vi "Sorting by.vi"(1 "Queue":T1(array[cluster])=[{"Measure?"=TRUE, "Area (cm^2)"=0.0, "Cell Label"="", "Cell Description"="", "Cell Position"=0, "Time in rig (h)"=0.0, "Time to next scan (min)"=0.0, "Scan number"=0.0, "When did you stick it in?"=0.0, "Time between scans (min)"=0.0, "Time of the last scan(min)"=0.0, "Scan settings in queue"=0}, {"Measure?"=TRUE, "Area (cm^2)"=0.0, "Cell Label"="", "Cell Description"="", "Cell Position"=0, "Time in rig (h)"=0.0, "Time to next scan (min)"=0.0, "Scan number"=0.0, "When did you stick it in?"=0.0, "Time between scans (min)"=0.0, "Time of the last scan(min)"=0.0, "Scan settings in queue"=0}, {"Measure?"=TRUE, "Area (cm^2)"=0.0, "Cell Label"="", "Cell Description"="", "Cell Position"=0, "Time in rig (h)"=0.0, "Time to next scan (min)"=0.0, "Scan number"=0.0, "When did you stick it in?"=0.0, "Time between scans (min)"=0.0, "Time of the last scan(min)"=0.0, "Scan settings in queue"=0}, {"Measure?"=TRUE, "Area (cm^2)"=0.0, "Cell Label"="", "Cell Description"="", "Cell Position"=0, "Time in rig (h)"=0.0, "Time to next scan (min)"=0.0, "Scan number"=0.0, "When did you stick it in?"=0.0, "Time between scans (min)"=0.0, "Time of the last scan(min)"=0.0, "Scan settings in queue"=0}, {"Measure?"=TRUE, "Area (cm^2)"=0.0, "Cell Label"="", "Cell Description"="", "Cell Position"=0, "Time in rig (h)"=0.0, "Time to next scan (min)"=0.0, "Scan number"=0.0, "When did you stick it in?"=0.0, "Time between scans (min)"=0.0, "Time of the last scan(min)"=0.0, "Scan settings in queue"=0}, {"Measure?"=TRUE, "Area (cm^2)"=0.0, "Cell Label"="", "Cell Description"="", "Cell Position"=0, "Time in rig (h)"=0.0, "Time to next scan (min)"=0.0, "Scan number"=0.0, "When did you stick it in?"=0.0, "Time between scans (min)"=0.0, "Time of the last scan(min)"=0.0, "Scan settings in queue"=0}, {"Measure?"=TRUE, "Area (cm^2)"=0.0, "Cell Label"="", "Cell Description"="", "Cell Position"=0, "Time in rig (h)"=0.0, "Time to next scan (min)"=0.0, "Scan number"=0.0, "When did you stick it in?"=0.0, "Time between scans (min)"=0.0, "Time of the last scan(min)"=0.0, "Scan settings in queue"=0}, {"Measure?"=TRUE, "Area (cm^2)"=0.0, "Cell Label"="", "Cell Description"="", "Cell Position"=0, "Time in rig (h)"=0.0, "Time to next scan (min)"=0.0, "Scan number"=0.0, "When did you stick it in?"=0.0, "Time between scans (min)"=0.0, "Time of the last scan(min)"=0.0, "Scan settings in queue"=0}, {"Measure?"=TRUE, "Area (cm^2)"=0.0, "Cell Label"="", "Cell Description"="", "Cell Position"=0, "Time in rig (h)"=0.0, "Time to next scan (min)"=0.0, "Scan number"=0.0, "When did you stick it in?"=0.0, "Time between scans (min)"=0.0, "Time of the last scan(min)"=0.0, "Scan settings in queue"=0}, {"Measure?"=TRUE, "Area (cm^2)"=0.0, "Cell Label"="", "Cell Description"="", "Cell Position"=0, "Time in rig (h)"=0.0, "Time to next scan (min)"=0.0, "Scan number"=0.0, "When did you stick it in?"=0.0, "Time between scans (min)"=0.0, "Time of the last scan(min)"=0.0, "Scan settings in queue"=0}, {"Measure?"=TRUE, "Area (cm^2)"=0.0, "Cell Label"="", "Cell Description"="", "Cell Position"=0, "Time in rig (h)"=0.0, "Time to next scan (min)"=0.0, "Scan number"=0.0, "When did you stick it in?"=0.0, "Time between scans (min)"=0.0, "Time of the last scan(min)"=0.0, "Scan settings in queue"=0}, {"Measure?"=TRUE, "Area (cm^2)"=0.0, "Cell Label"="", "Cell Description"="", "Cell Position"=0, "Time in rig (h)"=0.0, "Time to next scan (min)"=0.0, "Scan number"=0.0, "When did you stick it in?"=0.0, "Time between scans (min)"=0.0, "Time of the last scan(min)"=0.0, "Scan settings in queue"=0}, {"Measure?"=TRUE, "Area (cm^2)"=0.0, "Cell Label"="", "Cell Description"="", "Cell Position"=0, "Time in rig (h)"=0.0, "Time to next scan (min)"=0.0, "Scan number"=0.0, "When did you stick it in?"=0.0, "Time between scans (min)"=0.0, "Time of the last scan(min)"=0.0, "Scan settings in queue"=0}, {"Measure?"=TRUE, "Area (cm^2)"=0.0, "Cell Label"="", "Cell Description"="", "Cell Position"=0, "Time in rig (h)"=0.0, "Time to next scan (min)"=0.0, "Scan number"=0.0, "When did you stick it in?"=0.0, "Time between scans (min)"=0.0, "Time of the last scan(min)"=0.0, "Scan settings in queue"=0}, {"Measure?"=TRUE, "Area (cm^2)"=0.0, "Cell Label"="", "Cell Description"="", "Cell Position"=0, "Time in rig (h)"=0.0, "Time to next scan (min)"=0.0, "Scan number"=0.0, "When did you stick it in?"=0.0, "Time between scans (min)"=0.0, "Time of the last scan(min)"=0.0, "Scan settings in queue"=0}, {"Measure?"=TRUE, "Area (cm^2)"=0.0, "Cell Label"="", "Cell Description"="", "Cell Position"=0, "Time in rig (h)"=0.0, "Time to next scan (min)"=0.0, "Scan number"=0.0, "When did you stick it in?"=0.0, "Time between scans (min)"=0.0, "Time of the last scan(min)"=0.0, "Scan settings in queue"=0}] {"Scan settings in queue" items=["Regular", "Inverted"]; "Time of the last scan(min)" format="%<%H:%M:%S>t"; "When did you stick it in?" format="%<%H:%M:%S>t"; "Time to next scan (min)" format="%<%H:%M:%S>t"; "Time in rig (h)" format="%<%H:%M:%S>t"}, 2 "Sort by":u16(ring) items=["Cell position", "Cell label", "Time in rig"]) -> (0 "Queue 2":T1(array[cluster])=[{"Measure?"=TRUE, "Area (cm^2)"=0.0, "Cell Label"="", "Cell Description"="", "Cell Position"=0, "Time in rig (h)"=0.0, "Time to next scan (min)"=0.0, "Scan number"=0.0, "When did you stick it in?"=0.0, "Time between scans (min)"=0.0, "Time of the last scan(min)"=0.0, "Scan settings in queue"=0}, {"Measure?"=TRUE, "Area (cm^2)"=0.0, "Cell Label"="", "Cell Description"="", "Cell Position"=0, "Time in rig (h)"=0.0, "Time to next scan (min)"=0.0, "Scan number"=0.0, "When did you stick it in?"=0.0, "Time between scans (min)"=0.0, "Time of the last scan(min)"=0.0, "Scan settings in queue"=0}, {"Measure?"=TRUE, "Area (cm^2)"=0.0, "Cell Label"="", "Cell Description"="", "Cell Position"=0, "Time in rig (h)"=0.0, "Time to next scan (min)"=0.0, "Scan number"=0.0, "When did you stick it in?"=0.0, "Time between scans (min)"=0.0, "Time of the last scan(min)"=0.0, "Scan settings in queue"=0}, {"Measure?"=TRUE, "Area (cm^2)"=0.0, "Cell Label"="", "Cell Description"="", "Cell Position"=0, "Time in rig (h)"=0.0, "Time to next scan (min)"=0.0, "Scan number"=0.0, "When did you stick it in?"=0.0, "Time between scans (min)"=0.0, "Time of the last scan(min)"=0.0, "Scan settings in queue"=0}, {"Measure?"=TRUE, "Area (cm^2)"=0.0, "Cell Label"="", "Cell Description"="", "Cell Position"=0, "Time in rig (h)"=0.0, "Time to next scan (min)"=0.0, "Scan number"=0.0, "When did you stick it in?"=0.0, "Time between scans (min)"=0.0, "Time of the last scan(min)"=0.0, "Scan settings in queue"=0}, {"Measure?"=TRUE, "Area (cm^2)"=0.0, "Cell Label"="", "Cell Description"="", "Cell Position"=0, "Time in rig (h)"=0.0, "Time to next scan (min)"=0.0, "Scan number"=0.0, "When did you stick it in?"=0.0, "Time between scans (min)"=0.0, "Time of the last scan(min)"=0.0, "Scan settings in queue"=0}, {"Measure?"=TRUE, "Area (cm^2)"=0.0, "Cell Label"="", "Cell Description"="", "Cell Position"=0, "Time in rig (h)"=0.0, "Time to next scan (min)"=0.0, "Scan number"=0.0, "When did you stick it in?"=0.0, "Time between scans (min)"=0.0, "Time of the last scan(min)"=0.0, "Scan settings in queue"=0}, {"Measure?"=TRUE, "Area (cm^2)"=0.0, "Cell Label"="", "Cell Description"="", "Cell Position"=0, "Time in rig (h)"=0.0, "Time to next scan (min)"=0.0, "Scan number"=0.0, "When did you stick it in?"=0.0, "Time between scans (min)"=0.0, "Time of the last scan(min)"=0.0, "Scan settings in queue"=0}, {"Measure?"=TRUE, "Area (cm^2)"=0.0, "Cell Label"="", "Cell Description"="", "Cell Position"=0, "Time in rig (h)"=0.0, "Time to next scan (min)"=0.0, "Scan number"=0.0, "When did you stick it in?"=0.0, "Time between scans (min)"=0.0, "Time of the last scan(min)"=0.0, "Scan settings in queue"=0}, {"Measure?"=TRUE, "Area (cm^2)"=0.0, "Cell Label"="", "Cell Description"="", "Cell Position"=0, "Time in rig (h)"=0.0, "Time to next scan (min)"=0.0, "Scan number"=0.0, "When did you stick it in?"=0.0, "Time between scans (min)"=0.0, "Time of the last scan(min)"=0.0, "Scan settings in queue"=0}, {"Measure?"=TRUE, "Area (cm^2)"=0.0, "Cell Label"="", "Cell Description"="", "Cell Position"=0, "Time in rig (h)"=0.0, "Time to next scan (min)"=0.0, "Scan number"=0.0, "When did you stick it in?"=0.0, "Time between scans (min)"=0.0, "Time of the last scan(min)"=0.0, "Scan settings in queue"=0}, {"Measure?"=TRUE, "Area (cm^2)"=0.0, "Cell Label"="", "Cell Description"="", "Cell Position"=0, "Time in rig (h)"=0.0, "Time to next scan (min)"=0.0, "Scan number"=0.0, "When did you stick it in?"=0.0, "Time between scans (min)"=0.0, "Time of the last scan(min)"=0.0, "Scan settings in queue"=0}, {"Measure?"=TRUE, "Area (cm^2)"=0.0, "Cell Label"="", "Cell Description"="", "Cell Position"=0, "Time in rig (h)"=0.0, "Time to next scan (min)"=0.0, "Scan number"=0.0, "When did you stick it in?"=0.0, "Time between scans (min)"=0.0, "Time of the last scan(min)"=0.0, "Scan settings in queue"=0}, {"Measure?"=TRUE, "Area (cm^2)"=0.0, "Cell Label"="", "Cell Description"="", "Cell Position"=0, "Time in rig (h)"=0.0, "Time to next scan (min)"=0.0, "Scan number"=0.0, "When did you stick it in?"=0.0, "Time between scans (min)"=0.0, "Time of the last scan(min)"=0.0, "Scan settings in queue"=0}, {"Measure?"=TRUE, "Area (cm^2)"=0.0, "Cell Label"="", "Cell Description"="", "Cell Position"=0, "Time in rig (h)"=0.0, "Time to next scan (min)"=0.0, "Scan number"=0.0, "When did you stick it in?"=0.0, "Time between scans (min)"=0.0, "Time of the last scan(min)"=0.0, "Scan settings in queue"=0}, {"Measure?"=TRUE, "Area (cm^2)"=0.0, "Cell Label"="", "Cell Description"="", "Cell Position"=0, "Time in rig (h)"=0.0, "Time to next scan (min)"=0.0, "Scan number"=0.0, "When did you stick it in?"=0.0, "Time between scans (min)"=0.0, "Time of the last scan(min)"=0.0, "Scan settings in queue"=0}] {"Scan settings in queue" items=["Regular", "Inverted"]; "Time of the last scan(min)" format="%<%H:%M:%S>t"; "When did you stick it in?" format="%<%H:%M:%S>t"; "Time to next scan (min)" format="%<%H:%M:%S>t"; "Time in rig (h)" format="%<%H:%M:%S>t"})   [LabVIEW 2011]
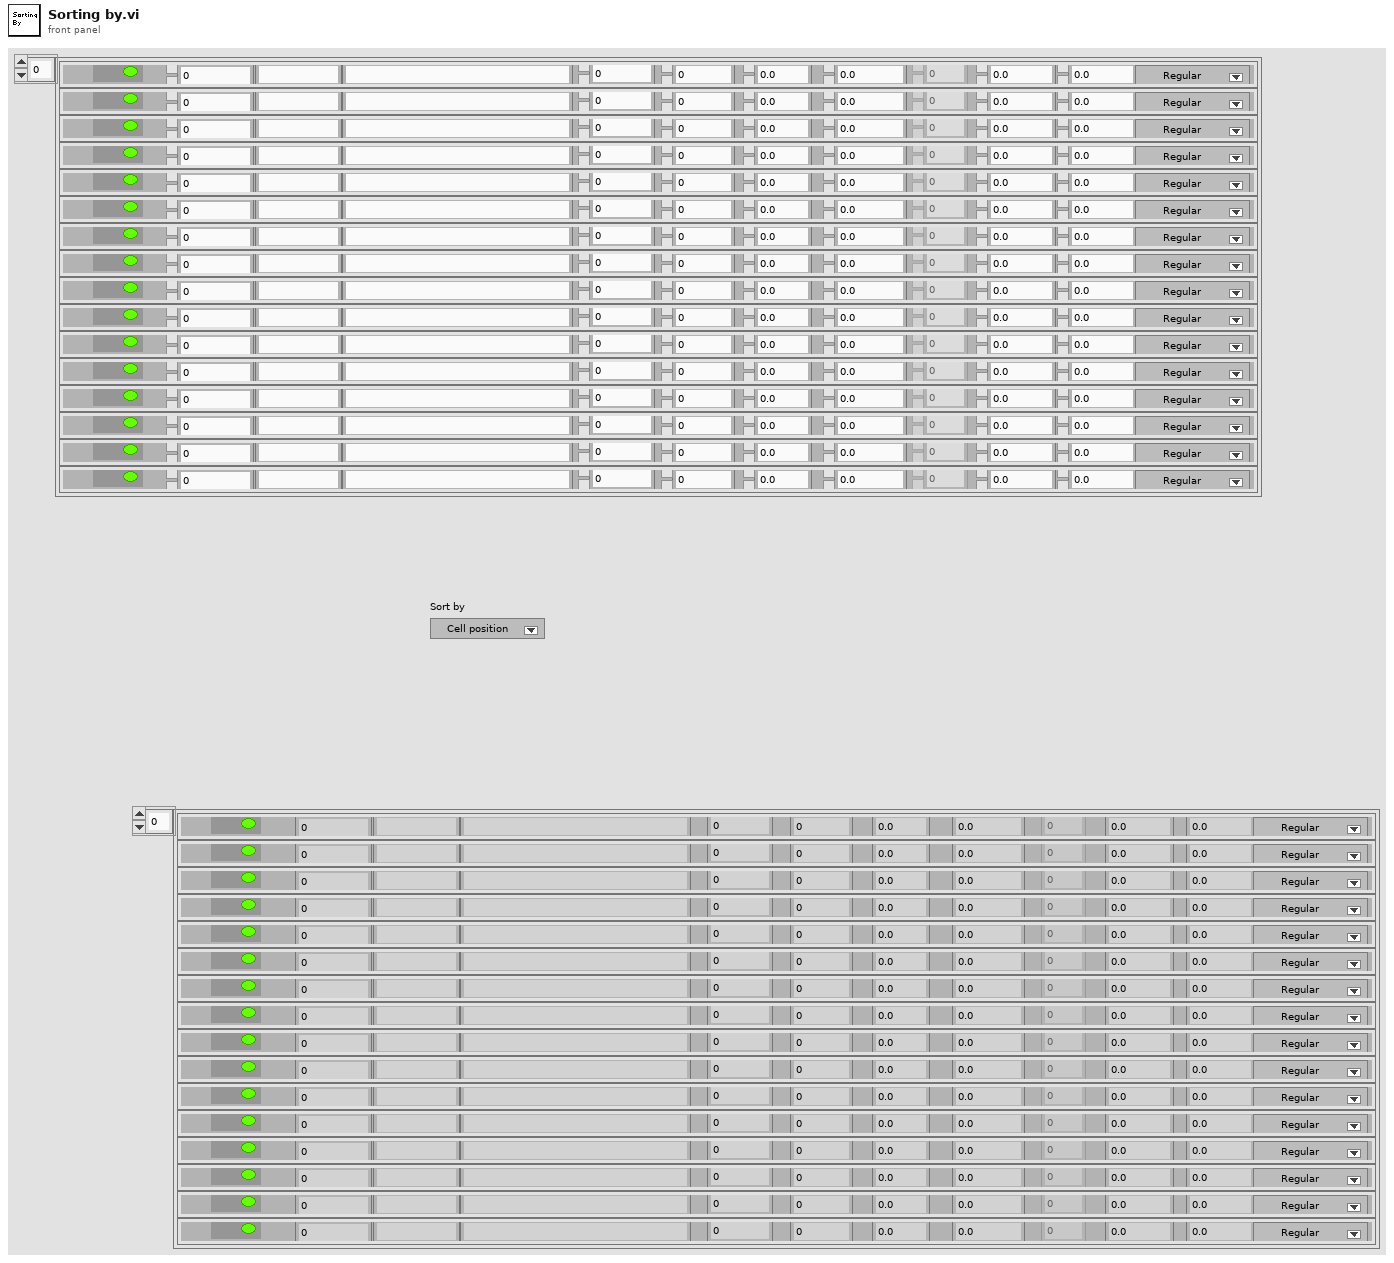
[diagram p1: front panel]
types:
  T1 = cluster{"Measure?":bool, "Area (cm^2)":dbl, "Cell Label":string, "Cell Description":string, "Cell Position":i32, "Time in rig (h)":dbl, "Time to next scan (min)":dbl, "Scan number":dbl, "When did you stick it in?":dbl, "Time between scans (min)":dbl, "Time of the last scan(min)":dbl, "Scan settings in queue":u16}[]
  T2 = cluster{"Measure?":bool, "Area (cm^2)":dbl, "Cell Label":string, "Cell Description":string, "Cell Position":i32, "Time in rig (h)":dbl, "Time to next scan (min)":dbl, "Scan number":dbl, "When did you stick it in?":dbl, "Time between scans (min)":dbl, "Time of the last scan(min)":dbl, "Scan settings in queue":u16}
  T3 = cluster{"cell label":string, "cell position":dbl}
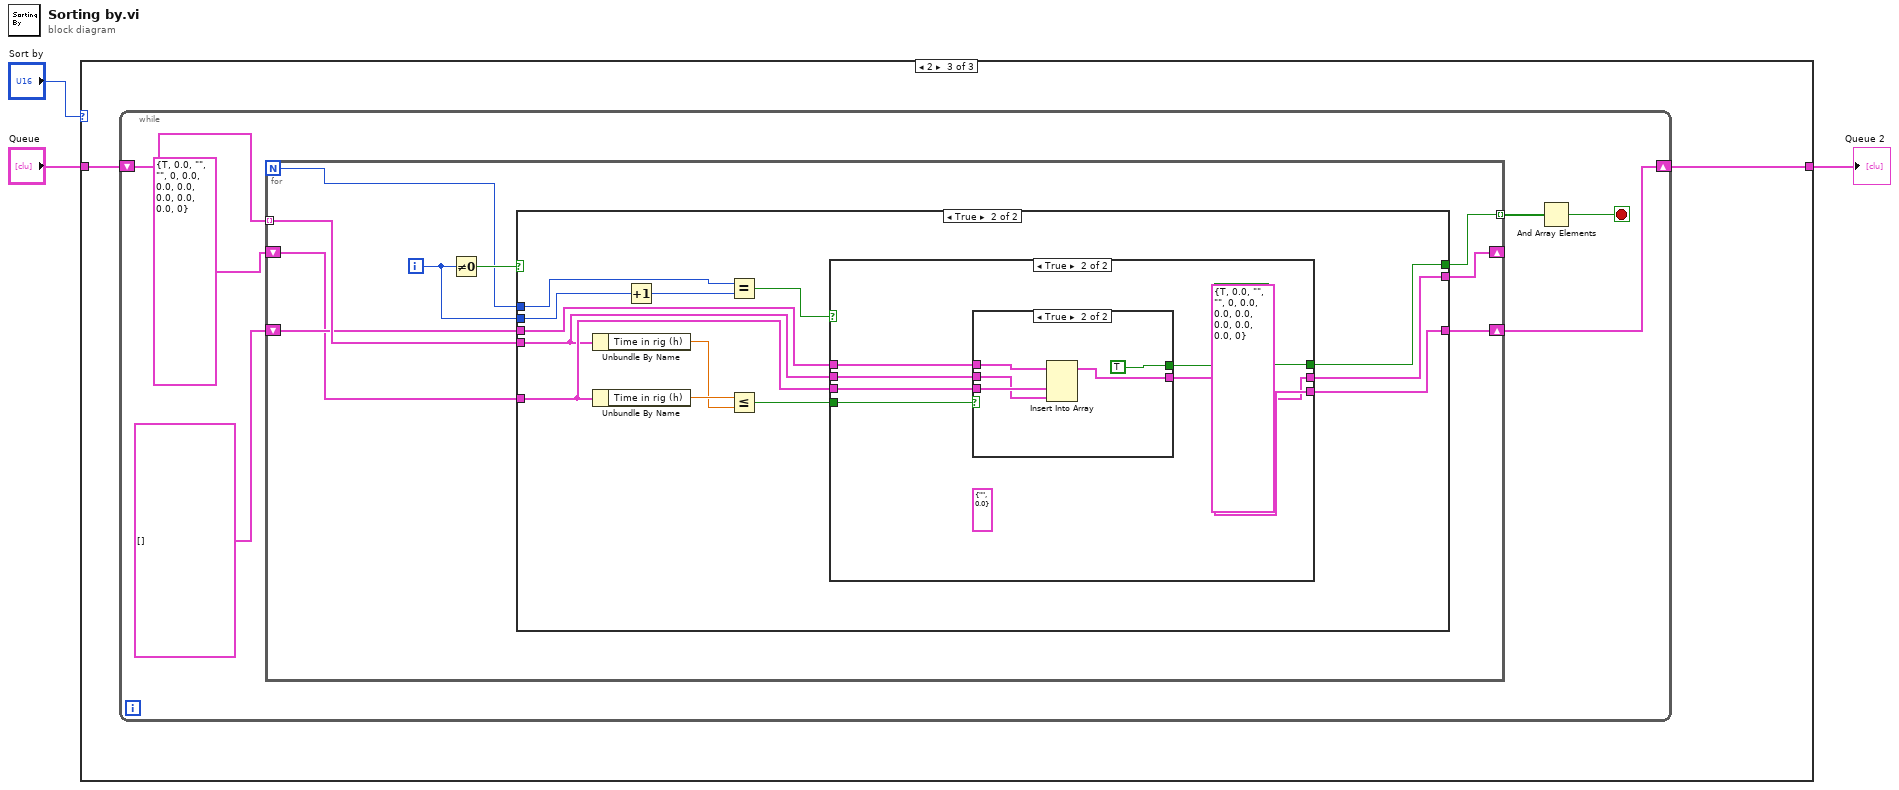
[diagram p0: block diagram]
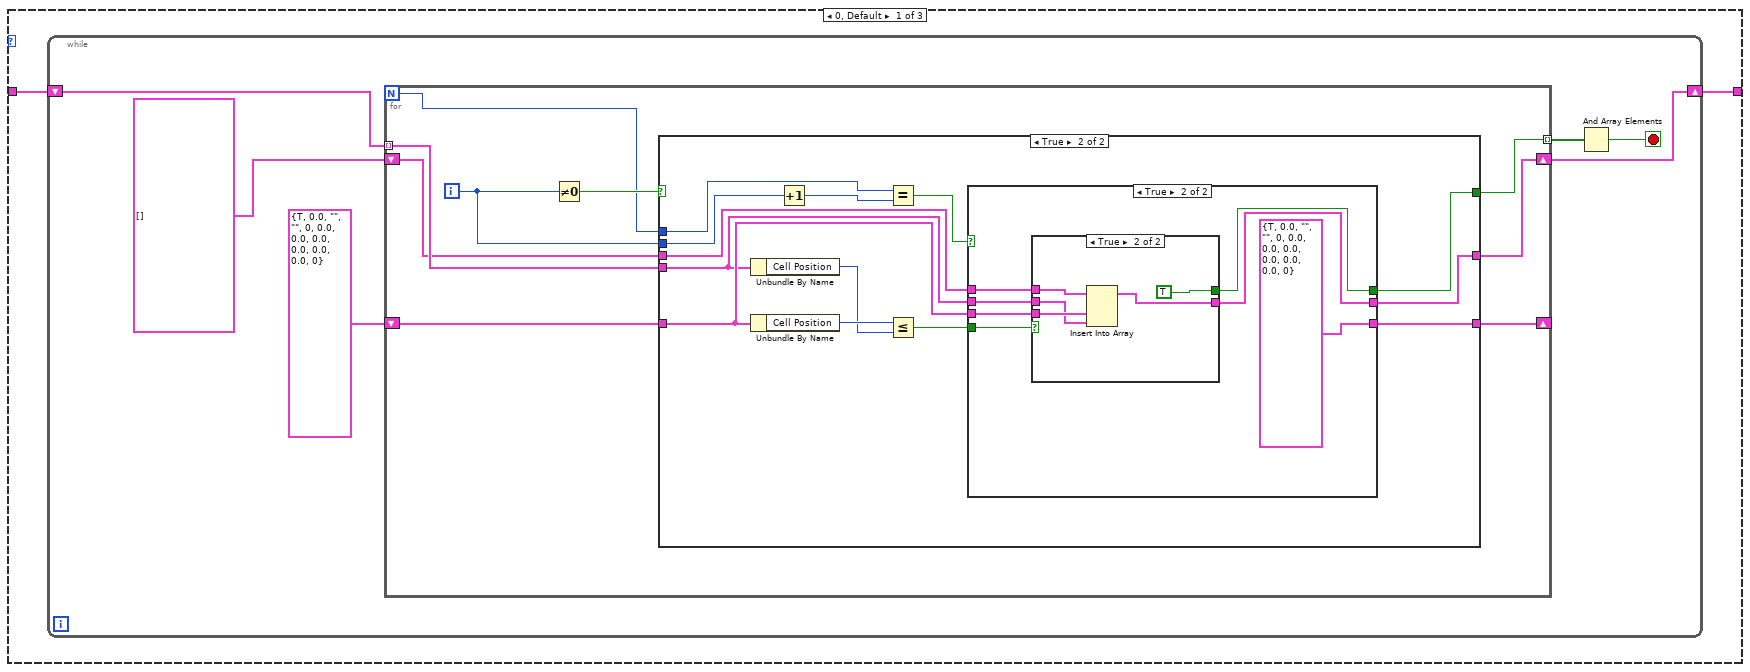
[diagram p2: hidden frame]
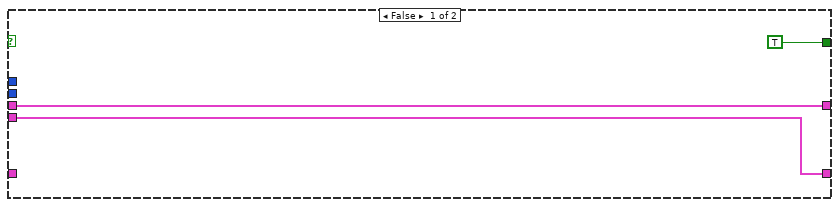
[diagram p3: hidden frame]
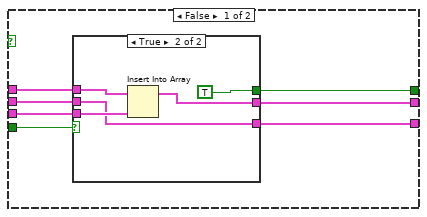
[diagram p4: hidden frame]
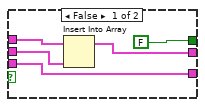
[diagram p5: hidden frame]
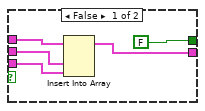
[diagram p6: hidden frame]
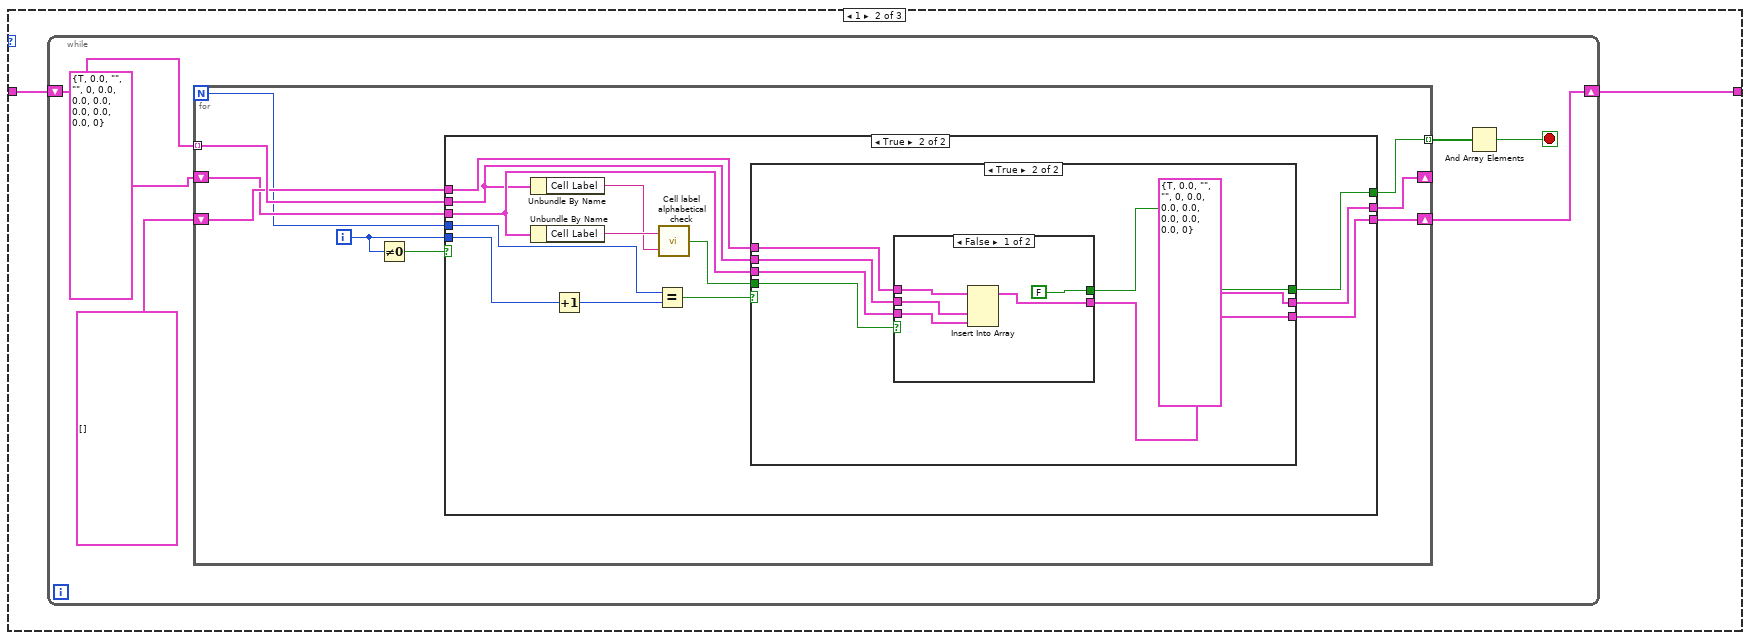
[diagram p7: hidden frame]
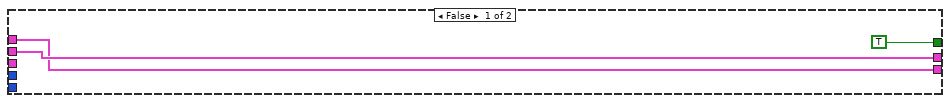
[diagram p8: hidden frame]
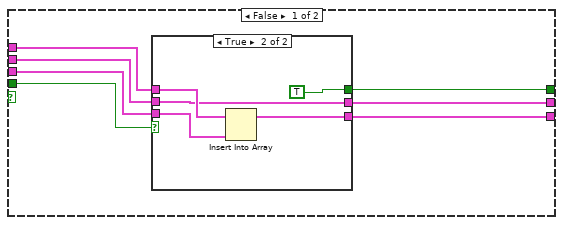
[diagram p9: hidden frame]
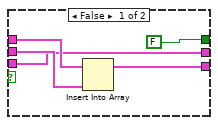
[diagram p10: hidden frame]
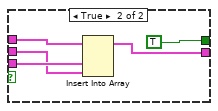
[diagram p11: hidden frame]
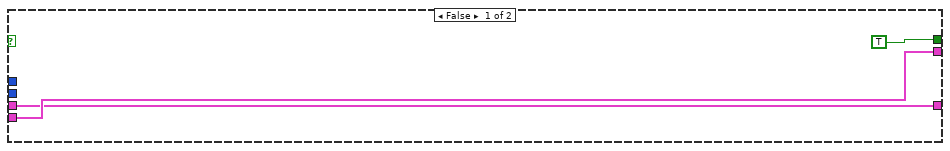
[diagram p12: hidden frame]
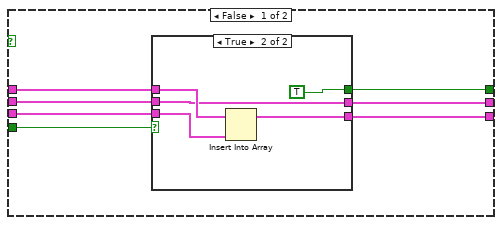
[diagram p13: hidden frame]
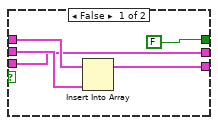
[diagram p14: hidden frame]
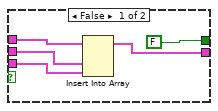
[diagram p15: hidden frame]
diagram:
  n1 = case shown="2" "Sort by" {
    tunnel: "Queue" -> [w5 w72 w139]
    tunnel: [w4 w71 w138] -> w1
    frame 0, Default {
      n2 = while {
        shift-right: [w11] -> w4
        shift-left: w5 -> [w10]
        stop <- w8 stop-if-true
        n3 = for {
          N -> [w13]
          tunnel: w10 -> [w20] mode=indexing
          shift-right: [w18] -> w11
          shift-left: T1 [] ("Queue") -> [w19]
          shift-right: [w15] -> _
          shift-left: T2 {"Measure?"=TRUE, "Area (cm^2)"=0.0, "Cell Label"="", "Cell Description"="", "Cell Position"=0, "Time in rig (h)"=0.0, "Time to next scan (min)"=0.0, "Scan number"=0.0, "When did you stick it in?"=0.0, "Time between scans (min)"=0.0, "Time of the last scan(min)"=0.0, "Scan settings in queue"=0} ("Cluster") -> [w17]
          tunnel: [w14] -> w9 mode=indexing
          i -> [w12]
          n4 = Not Equal To 0?(x=w12) -> (x != 0?=w16:bool)
          n5 = case shown="True" w16 {
            tunnel: w20 -> [w23 w29]
            tunnel: w19 -> [w22 w36]
            tunnel: [w22 w35] -> w18
            tunnel: w17 -> [_ w31]
            tunnel: [w23 w30] -> w15
            tunnel: [TRUE w28] -> w14
            tunnel: w13 -> [_ w27]
            tunnel: w12 -> [_ w25]
            frame False {
            }
            frame True {
              n6 = Unbundle By Name(w29) -> ("Cell Position"=w32:i32)
              n7 = Unbundle By Name(w31) -> ("Cell Position"=w33:i32)
              n8 = Increment(x=w25) -> (x+1=w26:i32)
              n9 = Equal?(x=w27, y=w26) -> (x = y?=w24:bool)
              n10 = Less Or Equal?(x=w33, y=w32) -> (x <= y?=w34:bool)
              n11 = case shown="True" w24 {
                tunnel: w36 -> [w43 w59]
                tunnel: [w42 w58] -> w35
                tunnel: w34 -> [w41 w60]
                tunnel: w31 -> [w40 w57]
                tunnel: [w39 T2 {"Measure?"=TRUE, "Area (cm^2)"=0.0, "Cell Label"="", "Cell Description"="", "Cell Position"=0, "Time in rig (h)"=0.0, "Time to next scan (min)"=0.0, "Scan number"=0.0, "When did you stick it in?"=0.0, "Time between scans (min)"=0.0, "Time of the last scan(min)"=0.0, "Scan settings in queue"=0} ("Cluster")] -> w30
                tunnel: w29 -> [w38 w56]
                tunnel: [w37 w55] -> w28
                frame False {
                  n12 = case shown="True" w41 {
                    tunnel: w43 -> [w48 w53]
                    tunnel: [w47 w52] -> w42
                    tunnel: w40 -> [w45 w51]
                    tunnel: [w45 w50] -> w39
                    tunnel: w38 -> [w46 w50]
                    tunnel: [FALSE TRUE] -> w37
                    frame False {
                      n13 = Insert Into Array(array=w48, new element=w46) -> (w47:T1)  [unwired: 1 in]
                    }
                    frame True {
                      n14 = Insert Into Array(array=w53, new element=w51) -> (w52:T1)  [unwired: 1 in]
                    }
                  }
                }
                frame True {
                  n15 = case shown="True" w60 {
                    tunnel: w59 -> [w64 w70]
                    tunnel: [w65 w69] -> w58
                    tunnel: w57 -> [w61 w68]
                    tunnel: w56 -> [w62 w67]
                    tunnel: [FALSE TRUE] -> w55
                    frame False {
                      n16 = Insert Into Array(array=w64, new element #1=w62, new element #2=w61) -> (w65:T1)  [unwired: 1 in]
                    }
                    frame True {
                      n17 = Insert Into Array(array=w70, new element #1=w68, new element #2=w67) -> (w69:T1)  [unwired: 1 in]
                    }
                  }
                }
              }
            }
          }
        }
        n18 = And Array Elements(Boolean array=w9) -> (logical AND=w8:bool)
      }
    }
    frame 1 {
      n19 = while {
        shift-right: [w78] -> w71
        shift-left: w72 -> [w77]
        stop <- w75 stop-if-true
        n20 = for {
          N -> [w80]
          tunnel: w77 -> [w87] mode=indexing
          shift-right: [w85] -> w78
          shift-left: T1 [] ("Queue") -> [w86]
          shift-right: [w82] -> _
          shift-left: T2 {"Measure?"=TRUE, "Area (cm^2)"=0.0, "Cell Label"="", "Cell Description"="", "Cell Position"=0, "Time in rig (h)"=0.0, "Time to next scan (min)"=0.0, "Scan number"=0.0, "When did you stick it in?"=0.0, "Time between scans (min)"=0.0, "Time of the last scan(min)"=0.0, "Scan settings in queue"=0} ("Cluster") -> [w84]
          tunnel: [w81] -> w76 mode=indexing
          i -> [w79]
          n21 = Not Equal To 0?(x=w79) -> (x != 0?=w83:bool)
          n22 = case shown="True" w83 {
            tunnel: w87 -> [w90 w96]
            tunnel: w86 -> [w89 w103]
            tunnel: [w89 w102] -> w85
            tunnel: w84 -> [_ w98]
            tunnel: [w90 w97] -> w82
            tunnel: [TRUE w95] -> w81
            tunnel: w80 -> [_ w94]
            tunnel: w79 -> [_ w92]
            frame False {
            }
            frame True {
              n23 = Unbundle By Name(w96) -> ("Cell Label"=w99:string)
              n24 = Unbundle By Name(w98) -> ("Cell Label"=w100:string)
              n25 = Increment(x=w92) -> (x+1=w93:i32)
              n26 = Equal?(x=w94, y=w93) -> (x = y?=w91:bool)
              n27 = call "Cell label  alphabetical check.vi"("Cell label 2"=w99, "Cell label 1"=w100) -> ("Is cell label 1 lower than cell label 2?"=w101:bool)
              n28 = case shown="True" w91 {
                tunnel: w103 -> [w110 w126]
                tunnel: [w109 w125] -> w102
                tunnel: w101 -> [w108 w127]
                tunnel: w98 -> [w107 w124]
                tunnel: [w106 T2 {"Measure?"=TRUE, "Area (cm^2)"=0.0, "Cell Label"="", "Cell Description"="", "Cell Position"=0, "Time in rig (h)"=0.0, "Time to next scan (min)"=0.0, "Scan number"=0.0, "When did you stick it in?"=0.0, "Time between scans (min)"=0.0, "Time of the last scan(min)"=0.0, "Scan settings in queue"=0} ("Cluster")] -> w97
                tunnel: w96 -> [w105 w123]
                tunnel: [w104 w122] -> w95
                frame False {
                  n29 = case shown="True" w108 {
                    tunnel: w110 -> [w115 w120]
                    tunnel: [w114 w119] -> w109
                    tunnel: w107 -> [w112 w118]
                    tunnel: [w112 w117] -> w106
                    tunnel: w105 -> [w113 w117]
                    tunnel: [FALSE TRUE] -> w104
                    frame False {
                      n30 = Insert Into Array(array=w115, new element=w113) -> (w114:T1)  [unwired: 1 in]
                    }
                    frame True {
                      n31 = Insert Into Array(array=w120, new element=w118) -> (w119:T1)  [unwired: 1 in]
                    }
                  }
                }
                frame True {
                  n32 = case shown="False" w127 {
                    tunnel: w126 -> [w131 w137]
                    tunnel: [w132 w136] -> w125
                    tunnel: w124 -> [w129 w135]
                    tunnel: w123 -> [w128 w134]
                    tunnel: [FALSE TRUE] -> w122
                    frame False {
                      n33 = Insert Into Array(array=w131, new element #1=w128, new element #2=w129) -> (w132:T1)  [unwired: 1 in]
                    }
                    frame True {
                      n34 = Insert Into Array(array=w137, new element #1=w135, new element #2=w134) -> (w136:T1)  [unwired: 1 in]
                    }
                  }
                }
              }
            }
          }
        }
        n35 = And Array Elements(Boolean array=w76) -> (logical AND=w75:bool)
      }
    }
    frame 2 {
      n36 = while {
        shift-right: [w145] -> w138
        shift-left: w139 -> [w144]
        stop <- w142 stop-if-true
        n37 = for {
          N -> [w147]
          tunnel: w144 -> [w154] mode=indexing
          shift-right: [w152] -> w145
          shift-left: T1 [] ("Queue") -> [w153]
          shift-right: [w149] -> _
          shift-left: T2 {"Measure?"=TRUE, "Area (cm^2)"=0.0, "Cell Label"="", "Cell Description"="", "Cell Position"=0, "Time in rig (h)"=0.0, "Time to next scan (min)"=0.0, "Scan number"=0.0, "When did you stick it in?"=0.0, "Time between scans (min)"=0.0, "Time of the last scan(min)"=0.0, "Scan settings in queue"=0} ("Cluster") -> [w151]
          tunnel: [w148] -> w143 mode=indexing
          i -> [w146]
          n38 = Not Equal To 0?(x=w146) -> (x != 0?=w150:bool)
          n39 = case shown="True" w150 {
            tunnel: w154 -> [w157 w163]
            tunnel: w153 -> [w156 w170]
            tunnel: [w156 w169] -> w152
            tunnel: w151 -> [_ w165]
            tunnel: [w157 w164] -> w149
            tunnel: [TRUE w162] -> w148
            tunnel: w147 -> [_ w161]
            tunnel: w146 -> [_ w159]
            frame False {
            }
            frame True {
              n40 = Unbundle By Name(w163) -> ("Time in rig (h)"=w166:dbl)
              n41 = Unbundle By Name(w165) -> ("Time in rig (h)"=w167:dbl)
              n42 = Increment(x=w159) -> (x+1=w160:i32)
              n43 = Equal?(x=w161, y=w160) -> (x = y?=w158:bool)
              n44 = Less Or Equal?(x=w167, y=w166) -> (x <= y?=w168:bool)
              n45 = case shown="True" w158 {
                tunnel: w170 -> [w177 w193]
                tunnel: [w176 w192] -> w169
                tunnel: w168 -> [w175 w194]
                tunnel: w165 -> [w174 w191]
                tunnel: [w173 T2 {"Measure?"=TRUE, "Area (cm^2)"=0.0, "Cell Label"="", "Cell Description"="", "Cell Position"=0, "Time in rig (h)"=0.0, "Time to next scan (min)"=0.0, "Scan number"=0.0, "When did you stick it in?"=0.0, "Time between scans (min)"=0.0, "Time of the last scan(min)"=0.0, "Scan settings in queue"=0} ("Cluster")] -> w164
                tunnel: w163 -> [w172 w190]
                tunnel: [w171 w189] -> w162
                frame False {
                  n46 = case shown="True" w175 {
                    tunnel: w177 -> [w182 w187]
                    tunnel: [w181 w186] -> w176
                    tunnel: w174 -> [w179 w185]
                    tunnel: [w179 w184] -> w173
                    tunnel: w172 -> [w180 w184]
                    tunnel: [FALSE TRUE] -> w171
                    frame False {
                      n47 = Insert Into Array(array=w182, new element=w180) -> (w181:T1)  [unwired: 1 in]
                    }
                    frame True {
                      n48 = Insert Into Array(array=w187, new element=w185) -> (w186:T1)  [unwired: 1 in]
                    }
                  }
                }
                frame True {
                  (unwired) T3 {"cell label"="", "cell position"=0.0} ("Cluster")
                  n49 = case shown="True" w194 {
                    tunnel: w193 -> [w198 w204]
                    tunnel: [w199 w203] -> w192
                    tunnel: w191 -> [w195 w202]
                    tunnel: w190 -> [w196 w201]
                    tunnel: [FALSE TRUE] -> w189
                    frame False {
                      n50 = Insert Into Array(array=w198, new element #1=w196, new element #2=w195) -> (w199:T1)  [unwired: 1 in]
                    }
                    frame True {
                      n51 = Insert Into Array(array=w204, new element #1=w202, new element #2=w201) -> (w203:T1)  [unwired: 1 in]
                    }
                  }
                }
              }
            }
          }
        }
        n52 = And Array Elements(Boolean array=w143) -> (logical AND=w142:bool)
      }
    }
  }
  "Queue 2" <- w1
